vi "Diameter Tracing.vi"() -> ()   [LabVIEW 2011]
uses:
  <vilib>/vision/NI_Vision_Development_Module.lvlib
panel:
  out "selected path":path
  in  "Stop Updating Panel":bool
  in  "Search region offset (y)":dbl=70.0
  in  "Reference offset (y)":dbl=35.0
  in  "Calibration (1 pixel = ?um)":dbl=1.45
  out "Vessel Diameter":dbl[](graph)=[137.67987403869628]
  in  "Search region offset (x)":dbl=75.0
  out "Reference Image":T1(plugin-control)
  in  "Reference offset (x)":dbl=50.0
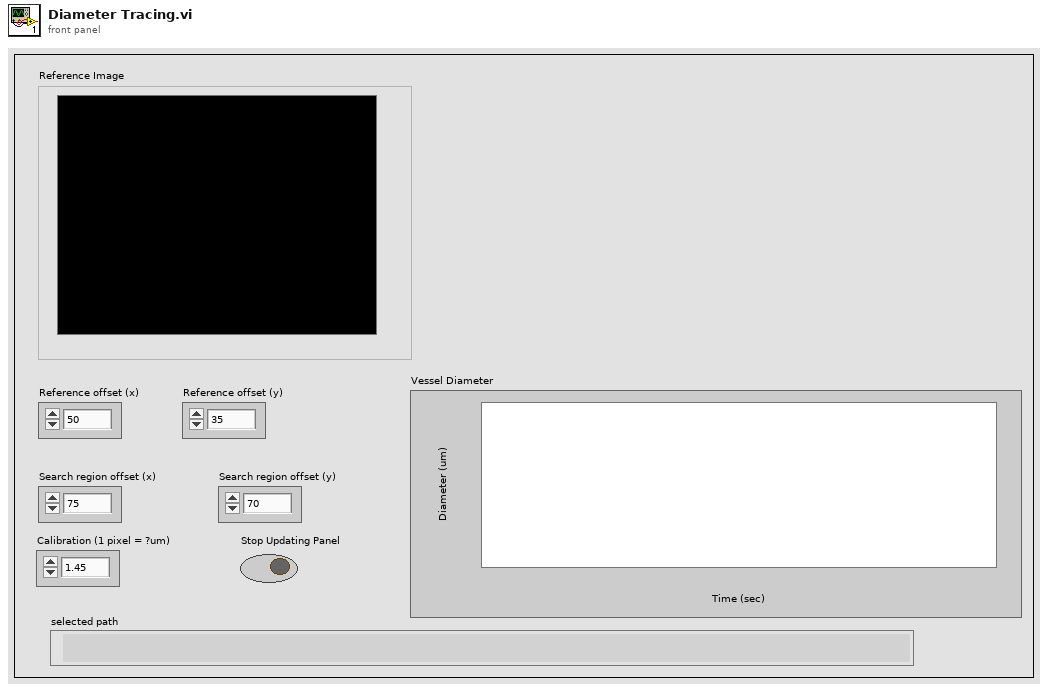
[diagram p1: front panel]
types:
  T1 = typedef "IMAQ Image.ctl" = refnum<image>
  T2 = typedef "Image Type" = u32
  T3 = typedef "AviRefnum.ctl" = refnum<k1>
  T4 = cluster{"width":u32, "height":u32, "framesPerSecond":u32, "compressionFilter":string, "hasData":bool}
  T5 = typedef "IMAQ Point" = cluster{"X":sgl, "Y":sgl}
  T6 = typedef "ROI Descriptor" = cluster{"Global Rectangle":i32[], "Contours":cluster{"ID":enum32{"External", "Internal"}, "Type":u32, "Coordinates":i32[]}[]}
  T7 = cluster{"Position":cluster{"x":sgl, "y":sgl}, "Angle":sgl, "Scale":sgl, "Score":sgl, "Bounding Box":cluster{"x":sgl, "y":sgl}[]}[]
  T8 = cluster{"Position":cluster{"x":sgl, "y":sgl}, "Position":cluster{"x":sgl, "y":sgl}}
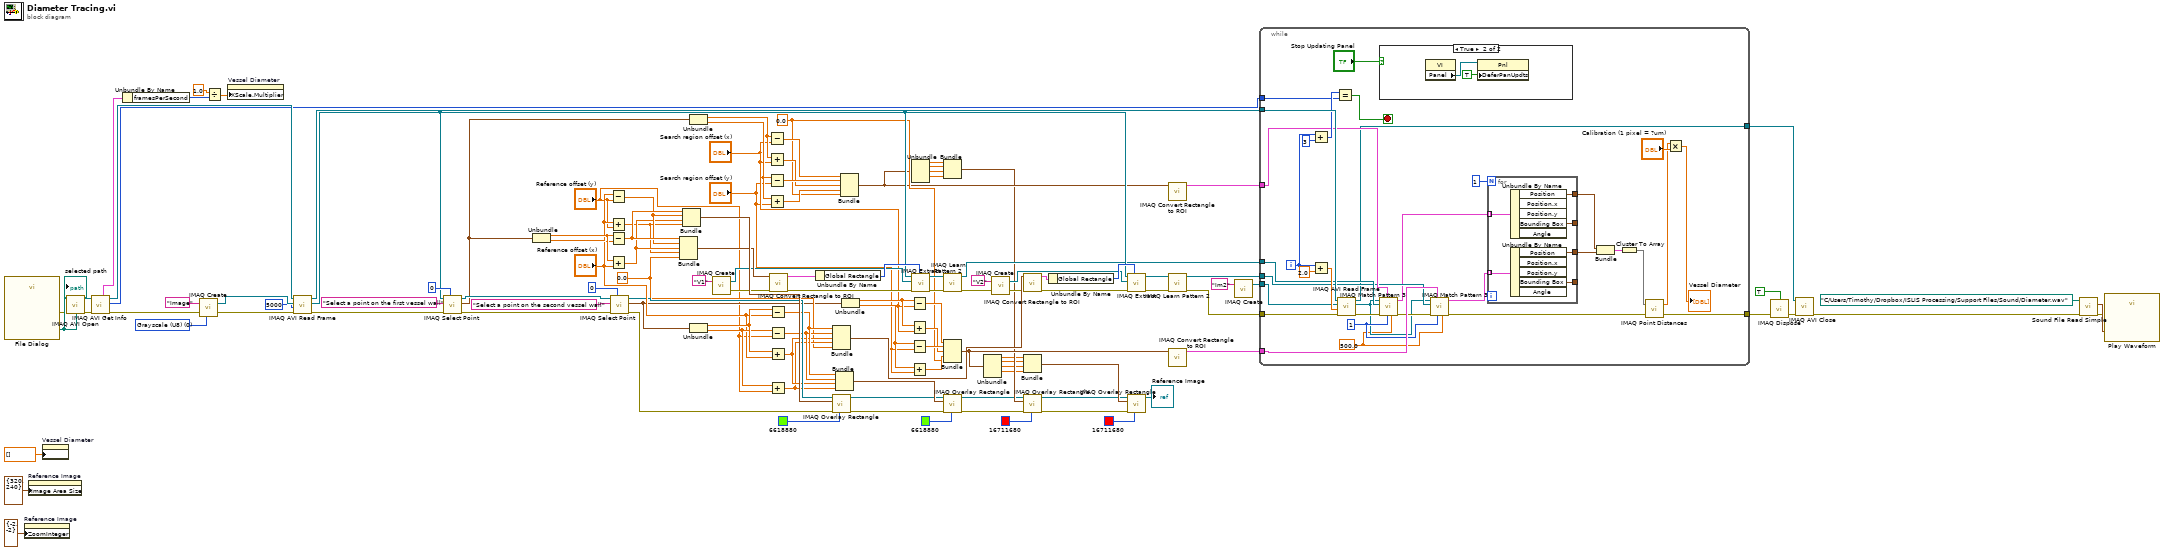
[diagram p0: block diagram]
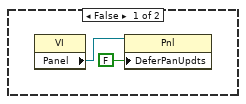
[diagram p2: hidden frame]
diagram:
  w47 = 0.0
  w82 = 0.0
  w115 = T2 0 items=["Grayscale (U8)", "Grayscale (I16)", "Grayscale (SGL)", "Complex (CSG)", "RGB (U32)", "HSL (U32)", "RGB (U64)", "Grayscale (U16)"] ("Image Type")
  n1 = call "File Dialog"() -> ("selected path"=w13:path, "error out"=w12:errorcluster)  [unwired: 12 in, 2 out]
  "selected path" <- w13
  n2 = property on="Reference Image" class="ImageControl"("ZoomInteger"=cluster{"X":i32, "Y":i32} {"X"=-2, "Y"=-2} ("ZoomInteger:All Elements")) -> ()  [unwired: 2 in, 2 out]
  n3 = property on="Reference Image" class="ImageControl"("Image Area Size"=cluster{"Width":u32, "Height":u32} {"Width"=320, "Height"=240} ("Image Area:Size:All Elements")) -> ()  [unwired: 2 in, 2 out]
  n4 = property on="Vessel Diameter" class="WFChart (strict)"("History Data"=dbl[] []) -> ()  [unwired: 2 in, 2 out]
  n5 = call "IMAQ AVI Open"("error in (no error)"=w12, "AVI Path"=w13) -> ("error out"=w121:errorcluster, "Avi Refnum"=w120:T3)  [unwired: 8 in]
  n6 = call "IMAQ AVI Get Info"("error in (no error)"=w121, "Avi Refnum"=w120) -> ("error out"=w118:errorcluster, "Number of Frames"=w63:u32, "Avi Refnum (duplicate)"=w113:T3, "Frame Data"=w20:T4)  [unwired: 5 in, 1 out]
  n7 = Unbundle By Name(w20) -> ("framesPerSecond"=w18:u32)
  n8 = call "IMAQ Create"("Image Name"="Image", "Image Type"=w115, "error in (no error)"=w118) -> ("New Image"=w117:T1, "error out"=w116:errorcluster)  [unwired: 2 in]
  n9 = Divide(x=1.0, y=w18) -> (x/y=w17:dbl)
  n10 = property on="Vessel Diameter" class="WFChart (strict)"("XScale.Multiplier"=w17) -> ()  [unwired: 2 in, 2 out]
  n11 = call "IMAQ AVI Read Frame"("error in (no error)"=w116, "Frame Number"=u32 5000, "Image"=w117, "Avi Refnum"=w113) -> ("error out"=w110:errorcluster, "Image Out"=w69:T1, "Avi Refnum (duplicate)"=w64:T3)  [unwired: 4 in, 1 out]
  n12 = call "IMAQ Select Point"("Window Number (0...15)"=0, "error in (no error)"=w110, "Prompt"="Select a point on the first vessel wall", "Image In"=w69) -> ("error out"=w108:errorcluster, "Point"=w49:T5, "Image Out (duplicate)"=w107:T1)  [unwired: 4 in, 1 out]
  n13 = Unbundle(w49) -> ("X"=w105:sgl, "Y"=w104:sgl)
  n14 = Subtract(x=w104, y="Reference offset (y)") -> (x-y=w91:dbl)
  n15 = Add(x=w104, y="Reference offset (y)") -> (x+y=w89:dbl)
  n16 = Subtract(x=w105, y="Reference offset (x)") -> (x-y=w92:dbl)
  n17 = Add(x=w105, y="Reference offset (x)") -> (x+y=w90:dbl)
  n18 = call "IMAQ Select Point"("Window Number (0...15)"=0, "error in (no error)"=w108, "Prompt"="Select a point on the second vessel wall", "Image In"=w107) -> ("error out"=w97:errorcluster, "Point"=w48:T5, "Image Out (duplicate)"=w94:T1)  [unwired: 4 in, 1 out]
  n19 = Bundle(w92, w91, w90, w89, w82) -> (w88:cluster{dbl, dbl, dbl, dbl, dbl})  [unwired: 1 in]
  n20 = Bundle(w92, w91, w90, w89) -> (w98:cluster{dbl, dbl, dbl, dbl})  [unwired: 1 in]
  n21 = Unbundle(w49) -> ("X"=w58:sgl, "Y"=w57:sgl)
  n22 = Unbundle(w48) -> ("X"=w103:sgl, "Y"=w102:sgl)
  n23 = call "IMAQ Create"("Image Name"="V1") -> ("New Image"=w71:T1, "error out"=w79:errorcluster)  [unwired: 4 in]
  n24 = Subtract(x=w58, y="Search region offset (x)") -> (x-y=w62:dbl)
  n25 = Add(x=w58, y="Search region offset (x)") -> (x+y=w60:dbl)
  n26 = Subtract(x=w57, y="Search region offset (y)") -> (x-y=w61:dbl)
  n27 = Add(x=w57, y="Search region offset (y)") -> (x+y=w59:dbl)
  n28 = Subtract(x=w103, y="Reference offset (x)") -> (x-y=w86:dbl)
  n29 = Subtract(x=w102, y="Reference offset (y)") -> (x-y=w85:dbl)
  n30 = Add(x=w103, y="Reference offset (x)") -> (x+y=w84:dbl)
  n31 = Add(x=w102, y="Reference offset (y)") -> (x+y=w83:dbl)
  n32 = call "IMAQ Convert Rectangle to ROI"("error in (no error)"=w79, "Rectangle"=w88) -> ("error out"=w72:errorcluster, "ROI Descriptor"=w75:T6)  [unwired: 7 in]
  n33 = Unbundle By Name(w75) -> ("Global Rectangle"=w74:i32[])
  n34 = call "IMAQ Overlay Rectangle"("Color"=u32 6618880, "error in (no error)"=w97, "Rectangle"=w98, "Image"=w94) -> ("error out"=w96:errorcluster, "Image Out"=w93:T1)  [unwired: 6 in]
  n35 = Bundle(w86, w85, w84, w83, w82) -> (w87:cluster{dbl, dbl, dbl, dbl, dbl})  [unwired: 1 in]
  n36 = Bundle(w86, w85, w84, w83) -> (w95:cluster{dbl, dbl, dbl, dbl})  [unwired: 1 in]
  n37 = Bundle(w62, w61, w60, w59, w47) -> (w38:cluster{dbl, dbl, dbl, dbl, dbl})  [unwired: 1 in]
  n38 = Unbundle(w48) -> ("X"=w52:sgl, "Y"=w51:sgl)
  n39 = Subtract(x=w52, y="Search region offset (x)") -> (x-y=w56:dbl)
  n40 = Add(x=w52, y="Search region offset (x)") -> (x+y=w54:dbl)
  n41 = Subtract(x=w51, y="Search region offset (y)") -> (x-y=w55:dbl)
  n42 = Add(x=w51, y="Search region offset (y)") -> (x+y=w53:dbl)
  n43 = Unbundle(w38) -> (w36:dbl, w35:dbl, w34:dbl, w33:dbl)  [unwired: 1 out]
  n44 = call "IMAQ Extract"("Optional Rectangle"=w74, "error in (no error)"=w72, "Image Dst"=w71, "Image Src"=w69) -> ("error out"=w68:errorcluster, "Image Dst Out"=w67:T1)  [unwired: 6 in]
  n45 = Bundle(w36, w35, w34, w33) -> (w32:cluster{dbl, dbl, dbl, dbl})  [unwired: 1 in]
  n46 = call "IMAQ Learn Pattern 2"("error in (no error)"=w68, "Image"=w67) -> ("error out"=w42:errorcluster, "Template Image Out"=w44:T1)  [unwired: 8 in]
  n47 = Bundle(w56, w55, w54, w53, w47) -> (w37:cluster{dbl, dbl, dbl, dbl, dbl})  [unwired: 1 in]
  n48 = call "IMAQ Overlay Rectangle"("Color"=u32 6618880, "error in (no error)"=w96, "Rectangle"=w95, "Image"=w93) -> ("error out"=w26:errorcluster, "Image Out"=w23:T1)  [unwired: 6 in]
  n49 = Unbundle(w37) -> (w31:dbl, w30:dbl, w29:dbl, w28:dbl)  [unwired: 1 out]
  n50 = call "IMAQ Create"("Image Name"="V2", "error in (no error)"=w42) -> ("New Image"=w70:T1, "error out"=w78:errorcluster)  [unwired: 3 in]
  n51 = call "IMAQ Convert Rectangle to ROI"("error in (no error)"=w78, "Rectangle"=w87) -> ("error out"=w73:errorcluster, "ROI Descriptor"=w77:T6)  [unwired: 7 in]
  n52 = Bundle(w31, w30, w29, w28) -> (w27:cluster{dbl, dbl, dbl, dbl})  [unwired: 1 in]
  n53 = call "IMAQ Overlay Rectangle"("Color"=u32 16711680, "error in (no error)"=w26, "Rectangle"=w32, "Image"=w23) -> ("error out"=w25:errorcluster, "Image Out"=w22:T1)  [unwired: 6 in]
  n54 = Unbundle By Name(w77) -> ("Global Rectangle"=w76:i32[])
  n55 = call "IMAQ Extract"("Optional Rectangle"=w76, "error in (no error)"=w73, "Image Dst"=w70, "Image Src"=w69) -> ("error out"=w66:errorcluster, "Image Dst Out"=w65:T1)  [unwired: 6 in]
  n56 = call "IMAQ Overlay Rectangle"("Color"=u32 16711680, "error in (no error)"=w25, "Rectangle"=w27, "Image"=w22) -> ("Image Out"=→"Reference Image":T1)  [unwired: 6 in, 1 out]
  n57 = call "IMAQ Convert Rectangle to ROI"("Rectangle"=w38) -> ("ROI Descriptor"=w46:T6)  [unwired: 8 in, 1 out]
  n58 = call "IMAQ Learn Pattern 2"("error in (no error)"=w66, "Image"=w65) -> ("error out"=w41:errorcluster, "Template Image Out"=w43:T1)  [unwired: 8 in]
  n59 = call "IMAQ Convert Rectangle to ROI"("Rectangle"=w37) -> ("ROI Descriptor"=w45:T6)  [unwired: 8 in, 1 out]
  n60 = call "IMAQ Create"("Image Name"="Im2") -> ("New Image"=w8:T1)  [unwired: 4 in, 1 out]
  n61 = while {
    tunnel: w64 -> [w154]
    tunnel: w63 -> [w148]
    tunnel: w46 -> [w146]
    tunnel: w45 -> [w145]
    tunnel: w44 -> [w142]
    tunnel: w43 -> [w141]
    tunnel: w41 -> [w140]
    tunnel: [w130] -> w21
    tunnel: w8 -> [w125]
    tunnel: [w122] -> w1
    i -> [w151]
    stop <- w147 stop-if-true
    w126 = sgl 500.0 ("Minimum Match Score")
    w139 = 1 ("Number of Matches Requested")
    n62 = Add(x=w151, y=3) -> (x+y=w149:i32)
    n63 = Add(x=w151, y=2.0) -> (x+y=w152:dbl)
    n64 = Equal?(x=w149, y=w148) -> (x = y?=w147:bool)
    n65 = call "IMAQ AVI Read Frame"("error in (no error)"=w140, "Frame Number"=w152, "Image"=w125, "Avi Refnum"=w154) -> ("error out"=w144:errorcluster, "Image Out"=w135:T1, "Avi Refnum (duplicate)"=w130:T3)  [unwired: 4 in, 1 out]
    n66 = case shown="True" "Stop Updating Panel" {
      frame False {
        n67 = property class="VI"() -> ("Panel"=w155:refnum<vi>)  [unwired: 2 in, 2 out]
        n68 = property class="Pnl"(reference=w155, "DeferPanUpdts"=FALSE ("Defer Panel Updates")) -> ()  [unwired: 1 in, 2 out]
      }
      frame True {
        n69 = property class="VI"() -> ("Panel"=w157:refnum<vi>)  [unwired: 2 in, 2 out]
        n70 = property class="Pnl"(reference=w157, "DeferPanUpdts"=TRUE ("Defer Panel Updates")) -> ()  [unwired: 1 in, 2 out]
      }
    }
    n71 = call "IMAQ Match Pattern 3"("Minimum Match Score"=w126, "Number of Matches Requested"=w139, "ROI Descriptor"=w146, "error in (no error)"=w144, "Template Image"=w142, "Image"=w135) -> ("error out"=w143:errorcluster, "Matches"=w137:T7)  [unwired: 3 in, 1 out]
    n72 = call "IMAQ Match Pattern 3"("Minimum Match Score"=w126, "Number of Matches Requested"=w139, "ROI Descriptor"=w145, "error in (no error)"=w143, "Template Image"=w141, "Image"=w135) -> ("error out"=w123:errorcluster, "Matches"=w136:T7)  [unwired: 3 in, 1 out]
    n73 = for {
      N: 1 -> [_]
      tunnel: w137 -> [w164] mode=indexing
      tunnel: w136 -> [w163] mode=indexing
      tunnel: [w162] -> _
      tunnel: [w161] -> _
      tunnel: [w160] -> w134
      tunnel: [w159] -> w133
      n74 = Unbundle By Name(w164) -> ("Position"=w160:cluster{"x":sgl, "y":sgl}, "Bounding Box"=w161:cluster{"x":sgl, "y":sgl}[])  [unwired: 3 out]
      n75 = Unbundle By Name(w163) -> ("Position"=w159:cluster{"x":sgl, "y":sgl}, "Bounding Box"=w162:cluster{"x":sgl, "y":sgl}[])  [unwired: 3 out]
    }
    n76 = Bundle("Position"=w134, "Position"=w133) -> (w131:T8)  [unwired: 1 in]
    n77 = Cluster To Array(cluster=w131) -> (array=w132:cluster{"x":sgl, "y":sgl}[])
    n78 = call "IMAQ Point Distances"("Points"=w132, "error in (no error)"=w123) -> ("Distances"=w128:sgl[], "error out"=w122:errorcluster)  [unwired: 3 in]
    n79 = Multiply(x=w128, y="Calibration (1 pixel = ?um)") -> (x*y=→"Vessel Diameter":dbl[])
  }
  n80 = call "IMAQ Dispose"("All Images? (No)"=TRUE, "error in (no error)"=w1) -> ("error out"=w7:errorcluster)  [unwired: 4 in]
  n81 = call "IMAQ AVI Close"("error in (no error)"=w7, "Avi Refnum"=w21) -> ("error out"=w3:errorcluster)  [unwired: 9 in]
  n82 = call <vilib>:"Sound File Read Simple.vi"("error in (no error)"=w3, "path"=path "C:/Users/Timothy/Dropbox/ISLIS Processing/Support Files/Sound/Diameter.wav") -> ("error out"=w4:errorcluster, "data"=w6:waveform(dbl)[])  [unwired: 6 in, 2 out]
  n83 = call "Play Waveform"("Data"=w6, "error in"=w4) -> ()  [unwired: 17 in, 1 out]
